vi "Delete Queue Mailbox.vi"(10 "Queue Mailbox":refnum<data-value>) -> (0 "error out":errorcluster)   [LabVIEW 2021, in "jettl.lvlib" / "Mailbox.lvlib"]
uses:
  Queue Mailbox/Queue Mailbox.lvclass
  Mailbox/Mailbox.lvlib
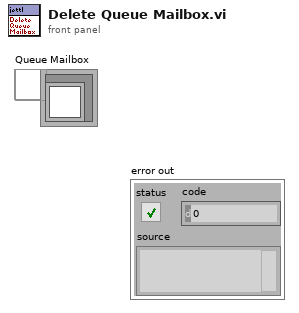
[diagram p1: front panel]
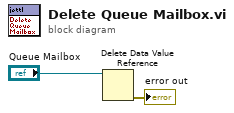
[diagram p0: block diagram]
diagram:
  n1 = Delete Data Value Reference(data value reference="Queue Mailbox") -> (error out=→"error out":errorcluster)  [unwired: 1 in, 1 out]
